vi "TwoDAQChannels_DifferentHardware_SingleGraph.vi"() -> ()   [LabVIEW 2019]
uses:
  <vilib>/DAQmx/read.llb/DAQmx Read (Analog 1D DBL 1Chan NSamp).vi
  <vilib>/DAQmx/create/channels.llb/DAQmx Create Channel (AI-Voltage-Basic).vi
  <vilib>/DAQmx/configure/timing.llb/DAQmx Timing (Sample Clock).vi
  <vilib>/DAQmx/miscellaneous.llb/DAQmx Fill In Error Info.vi
panel:
  out "error out 2":errorcluster
  out "error out":errorcluster
  out "XY Graph":cluster{cluster{dbl, "Waveform":dbl}[]}[](graph)
  in  "Stop":bool
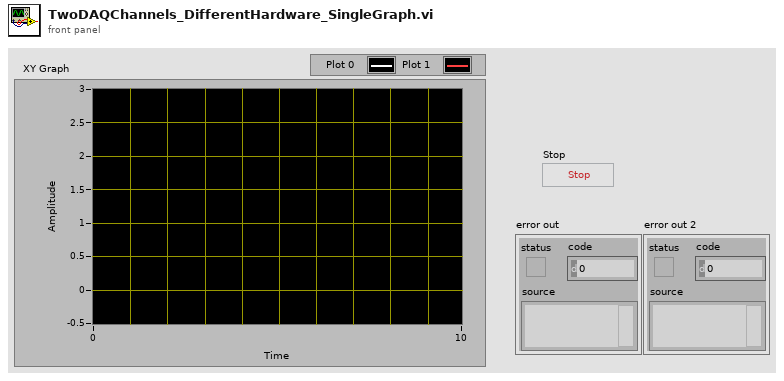
[diagram p1: front panel]
types:
  T1 = cluster{cluster{dbl, "Waveform":dbl}[], cluster{dbl, "Waveform":dbl}[], "Stop":bool}
  T2 = cluster{cluster{i32, "Waveform":dbl}[], cluster{dbl, "Waveform":dbl}[], "Stop":bool}
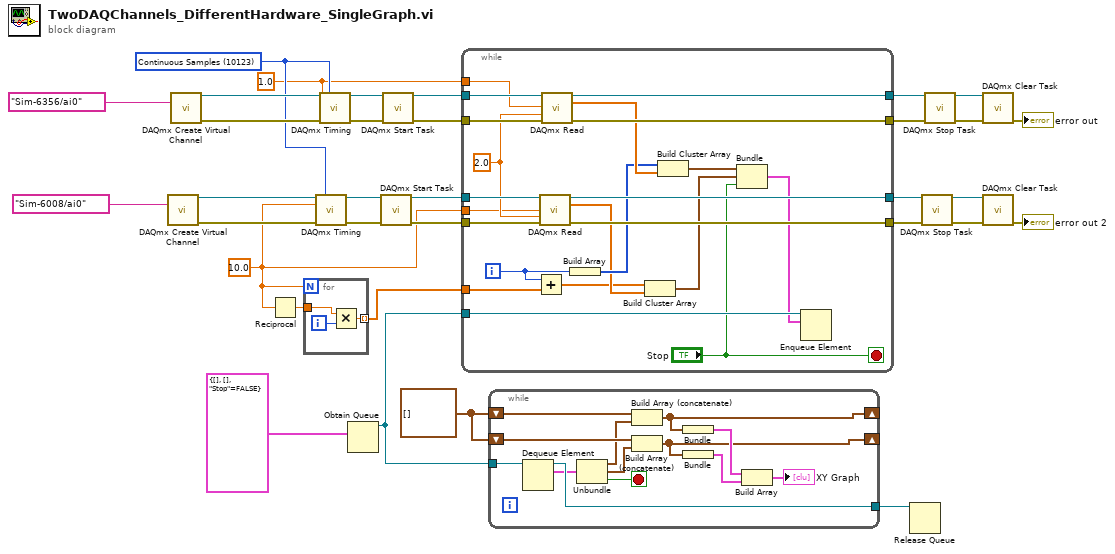
[diagram p0: block diagram]
diagram:
  w2 = cluster{dbl, "Waveform":dbl}[] []
  w15 = 10123 items=["Finite Samples"=10178, "Continuous Samples"=10123, "Hardware Timed Single Point"=12522] ("sample mode")
  w7 = 1.0 ("rate")
  w6 = 10.0 ("rate")
  n1 = call-poly <vilib>:"DAQmx Create Virtual Channel.vi"("physical channels"=tag "Sim-6008/ai0") -> ("task out"=w26:refnum<k21>, "error out"=w25:errorcluster)  [unwired: 13 in]
  n2 = call-poly <vilib>:"DAQmx Create Virtual Channel.vi"("physical channels"=tag "Sim-6356/ai0") -> ("task out"=w33:refnum<k21>, "error out"=w32:errorcluster)  [unwired: 13 in]
  n3 = Reciprocal(x=w6) -> (1/x=w5:dbl)
  n4 = for {
    N: w6 -> [_]
    tunnel: w5 -> [w36]
    tunnel: [w34] -> w4 mode=indexing
    i -> [w35]
    n5 = Multiply(x=w36, y=w35) -> (x*y=w34:dbl)
  }
  n6 = call-poly <vilib>:"DAQmx Timing.vi"("task/channels in"=w26, "sample mode"=w15, "rate"=w6, "error in"=w25) -> ("task out"=w10:refnum<k21>, "error out"=w24:errorcluster)  [unwired: 10 in]
  n7 = call-poly <vilib>:"DAQmx Timing.vi"("task/channels in"=w33, "sample mode"=w15, "rate"=w7, "error in"=w32) -> ("task out"=w13:refnum<k21>, "error out"=w31:errorcluster)  [unwired: 10 in]
  n8 = Obtain Queue(element data type=T1 {[], [], "Stop"=FALSE} ("output cluster")) -> (queue out=w8:refnum<queue>)  [unwired: 4 in, 2 out]
  n9 = call <vilib>:"DAQmx Start Task.vi"("task/channels in"=w10, "error in"=w24) -> ("task out"=w9:refnum<k21>, "error out"=w11:errorcluster)  [unwired: 12 in]
  n10 = call <vilib>:"DAQmx Start Task.vi"("task/channels in"=w13, "error in"=w31) -> ("task out"=w12:refnum<k21>, "error out"=w14:errorcluster)  [unwired: 12 in]
  n11 = while {
    tunnel: w12 -> [w58]
    tunnel: w14 -> [w57]
    tunnel: [w56] -> w30
    tunnel: [w55] -> w29
    tunnel: w9 -> [w54]
    tunnel: w11 -> [w53]
    tunnel: [w52] -> w23
    tunnel: [w51] -> w22
    tunnel: w8 -> [w49]
    tunnel: w7 -> [w47]
    tunnel: w6 -> [w46]
    tunnel: w4 -> [w42]
    i -> [w45]
    stop <- "Stop" stop-if-true
    w50 = 2.0 ("timeout")
    n12 = Add(x=w45, y=w42) -> (x+y=w41:dbl[])
    n13 = call-poly <vilib>:"DAQmx Read.vi"("task/channels in"=w54, "number of samples per channel"=w46, "timeout"=w50, "error in"=w53) -> ("task out"=w52:refnum<k21>, "data"=w43:dbl[], "error out"=w51:errorcluster)  [unwired: 9 in]
    n14 = call-poly <vilib>:"DAQmx Read.vi"("task/channels in"=w58, "number of samples per channel"=w47, "timeout"=w50, "error in"=w57) -> ("task out"=w56:refnum<k21>, "data"=w48:dbl[], "error out"=w55:errorcluster)  [unwired: 9 in]
    n15 = Build Array(w45) -> (w44:i32[])
    n16 = Build Cluster Array(w41, w43) -> (w40:cluster{dbl, "Waveform":dbl}[])
    n17 = Build Cluster Array(w44, w48) -> (w39:cluster{i32, "Waveform":dbl}[])
    n18 = Bundle(w39, w40, "Stop"="Stop") -> (w37:T2)  [unwired: 1 in]
    n19 = Enqueue Element(queue=w49, element=w37) -> ()  [unwired: 2 in, 3 out]
  }
  n20 = while {
    tunnel: w8 -> [w70]
    shift-right: [w59] -> _
    shift-left: w2 -> [w66]
    shift-right: [w65] -> _
    shift-left: w2 -> [w67]
    tunnel: [w71] -> w1
    stop <- w68 stop-if-true
    n21 = Dequeue Element(queue=w70) -> (queue out=w71:refnum<queue>, element=w69:T1)  [unwired: 2 in, 2 out]
    n22 = Unbundle(w69) -> (w61:cluster{dbl, "Waveform":dbl}[], w60:cluster{dbl, "Waveform":dbl}[], "Stop"=w68:bool)
    n23 = Build Array (concatenate)(w67, w61) -> (w65:cluster{dbl, "Waveform":dbl}[])
    n24 = Build Array (concatenate)(w66, w60) -> (w59:cluster{dbl, "Waveform":dbl}[])
    n25 = Bundle(w65) -> (w64:cluster{cluster{dbl, "Waveform":dbl}[]})  [unwired: 1 in]
    n26 = Bundle(w59) -> (w62:cluster{cluster{dbl, "Waveform":dbl}[]})  [unwired: 1 in]
    n27 = Build Array(w64, w62) -> (→"XY Graph":cluster{cluster{dbl, "Waveform":dbl}[]}[])
  }
  n28 = Release Queue(queue=w1) -> ()  [unwired: 2 in, 3 out]
  n29 = call <vilib>:"DAQmx Stop Task.vi"("task/channels in"=w23, "error in"=w22) -> ("task out"=w21:refnum<k21>, "error out"=w20:errorcluster)  [unwired: 12 in]
  n30 = call <vilib>:"DAQmx Stop Task.vi"("task/channels in"=w30, "error in"=w29) -> ("task out"=w28:refnum<k21>, "error out"=w27:errorcluster)  [unwired: 12 in]
  n31 = call <vilib>:"DAQmx Clear Task.vi"("task in"=w28, "error in"=w27) -> ("error out"=→"error out":errorcluster)  [unwired: 13 in]
  n32 = call <vilib>:"DAQmx Clear Task.vi"("task in"=w21, "error in"=w20) -> ("error out"=→"error out 2":errorcluster)  [unwired: 13 in]
